vi "identifyPortTypeWithFirstByte.vi"(1 "input_int":u8 format="%.0x") -> (0 "show_str_portType":string)   [LabVIEW 2011]
panel:
  # "本VI已经验证过下列对应关系        OK\nhex  decimal  portType\n03    3           SFP+\n\n11    17          QSFP+\n0D    13         QSFP+\n\n0F     15         HD\n10     16         HD\n14     20         HD\n15     21         HD"
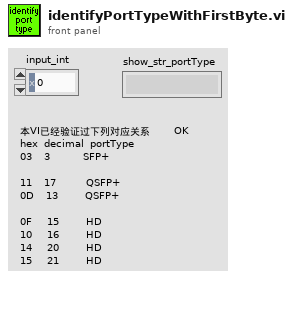
[diagram p1: front panel]
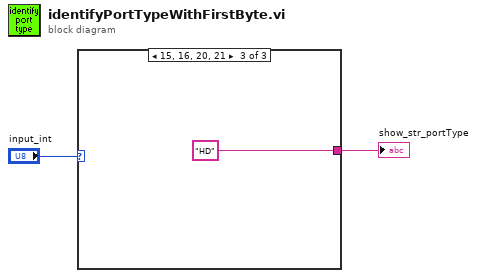
[diagram p0: block diagram]
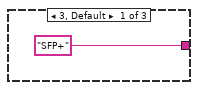
[diagram p2: hidden frame]
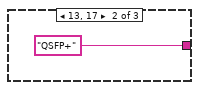
[diagram p3: hidden frame]
diagram:
  n1 = case shown="15, 16, 20, 21" "input_int" {
    tunnel: ["SFP+" "QSFP+" "HD"] -> w1
    frame 3, Default {
    }
    frame 13, 17 {
    }
    frame 15, 16, 20, 21 {
    }
  }
  "show_str_portType" <- w1
